vi "RunGlobalVI.vi"(8 "error in":errorcluster, 11 "VI input":refnum<vi>) -> (0 "error out":errorcluster)   [LabVIEW 2012, in "Spinner.xctl"]
uses:
  Spinner.xctl
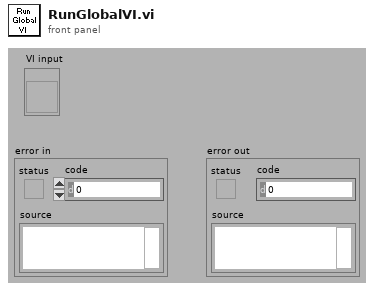
[diagram p1: front panel]
types:
  T1 = enum32{"Bad", "Idle", "Run top level", "Running"}
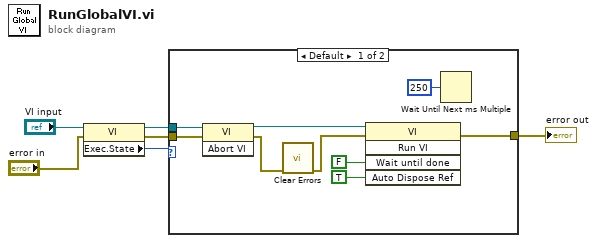
[diagram p0: block diagram]
diagram:
  n1 = property class="VI"(reference="VI input", error in="error in") -> (reference out=w5:refnum<vi>, error out=w4:errorcluster, "Exec.State"=w6:T1)
  n2 = case shown="Default" w6 {
    tunnel: w5 -> [w15 _]
    tunnel: w4 -> [w14 w16]
    tunnel: [w8 w16] -> w1
    frame Default {
      n3 = invoke class="VI" method="Abort VI"(reference=w15, error in=w14) -> (reference out=w13:refnum<vi>, error out=w10:errorcluster)  [unwired: 1 in, 1 out]
      n4 = call <vilib>:"Clear Errors.vi"("error in (no error)"=w10) -> ("error out"=w9:errorcluster)  [unwired: 6 in]
      n5 = invoke class="VI" method="Run VI"(reference=w13, error in=w9, "Wait until done"=FALSE ("Wait Until Done"), "Auto Dispose Ref"=TRUE ("Auto Dispose Reference")) -> (error out=w8:errorcluster)  [unwired: 1 in, 4 out]
      n6 = Wait Until Next ms Multiple(millisecond multiple=u32 250) -> ()  [unwired: 1 out]
    }
    frame "Run top level", "Running" {
    }
  }
  "error out" <- w1
